vi "datasource.initialize.vi"(8 "error in":errorcluster, 10 "Datasource Name":string, 11 "Nominal Client in":refnum<class "Nominal Client.lvclass">) -> (0 "error out":errorcluster, 2 "datasource rid":string, 3 "Nominal Client out":refnum<class "Nominal Client.lvclass">)   [LabVIEW 2024, in "nominal labview client.lvlib"]
uses:
  nominal labview client.lvlib
  <vilib>/Nominal/Nominal IO Client/Nominal Client/Nominal Client.lvclass
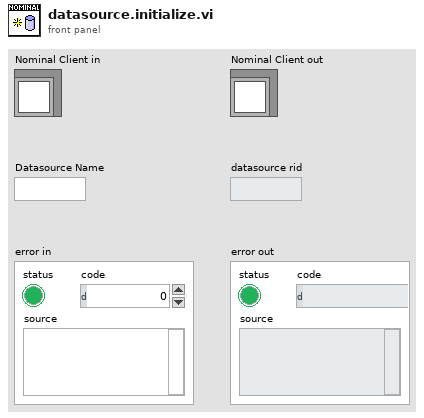
[diagram p1: front panel]
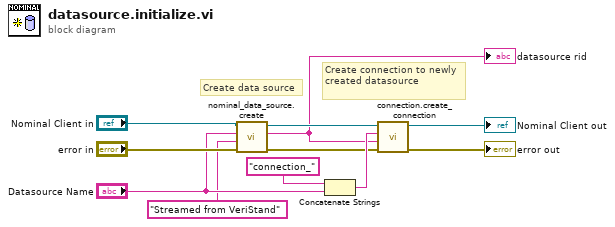
[diagram p0: block diagram]
diagram:
  # "Create connection to newly created datasource"
  # "Create data source"
  n1 = call <vilib>:"nominal_data_source.create.vi"("error in"="error in", "Description"="Streamed from VeriStand", "Name"="Datasource Name", "Nominal Client in"="Nominal Client in") -> ("error out"=w8:errorcluster, "rid"=w1:string, "Nominal Client out"=w9:refnum<class "Nominal Client.lvclass">)  [unwired: 4 in, 1 out]
  "datasource rid" <- w1
  n2 = Concatenate Strings("connection_" ("string"), "Datasource Name") -> (w11:string)
  n3 = call <vilib>:"connection.create_connection.vi"("error in"=w8, "nominalDataSourceRid"=w1, "name"=w11, "Nominal Client in"=w9) -> ("error out"=→"error out":errorcluster, "Nominal Client out"=→"Nominal Client out":refnum<class "Nominal Client.lvclass">)  [unwired: 4 in, 2 out]
